vi "Write DAQ VIEW.vi"(8 "error in (no error)":errorcluster, 10 "DAQ VIEW":refnum<class "base view.lvclass">, 11 "In":refnum<class "Recipe View.lvclass">) -> (0 "error out":errorcluster, 3 "Out":refnum<class "Recipe View.lvclass">)   [LabVIEW 2022 SP3, in "Recipe View.lvclass"]
uses:
  Recipe View.lvclass
  Recipe View.lvclass/Recipe View.ctl
  iView/base view/base view.lvclass
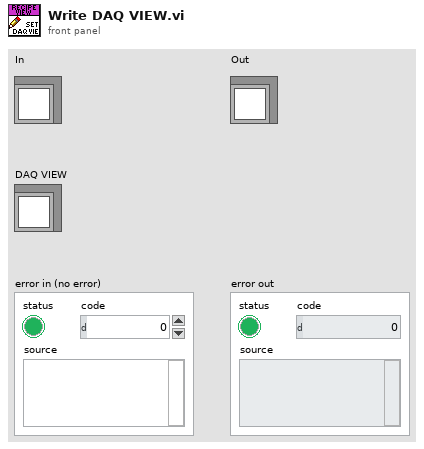
[diagram p1: front panel]
types:
  T1 = typedef "Recipe View.lvclass/Data.ctl" = cluster{"Recipe API.lvclass":refnum<class "Recipe API.lvclass">, "XY stage VIEW":refnum<class "base view.lvclass">, "Laser VIEW":refnum<class "base view.lvclass">, "Camera VIEW":refnum<class "base view.lvclass">, "DAQ VIEW":refnum<class "base view.lvclass">}
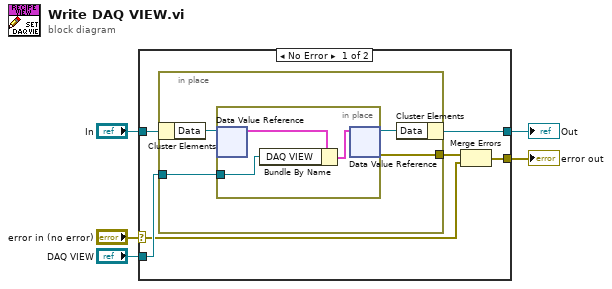
[diagram p0: block diagram]
diagram:
  n1 = case shown="No Error" "error in (no error)" {
    selector: "error in (no error)" -> [w6 w20]
    tunnel: [w7 w20] -> w4
    tunnel: [w11 w19] -> w3
    tunnel: "In" -> [w10 w19]
    tunnel: "DAQ VIEW" -> [w9 _]
    frame No Error {
      n2 = in-place {
        in-place-border: w9 -> [w13]
        in-place-border: [w12] -> w8
        n3 = in-place-cluster #1(w10) -> ("Data"=w14:refnum<data-value>)
        n4 = in-place {
          in-place-border: w13 -> [w17]
          n5 = in-place-dvr #2(w14) -> (w16:T1)  [unwired: 1 out]
          n6 = Bundle By Name(cluster=w16, "DAQ VIEW"=w17) -> (w18:T1)
          n7 = in-place-dvr #2(w18) -> (w15:refnum<data-value>, w12:errorcluster)
        }
        n8 = in-place-cluster #1("Data"=w15) -> (w11:refnum<class "Recipe View.lvclass">)
      }
      n9 = Merge Errors(w8, w6) -> (w7:errorcluster)
    }
    frame Error {
    }
  }
  "Out" <- w3
  "error out" <- w4
